vi "Store Executed Command.vi"(8 "error in (no error)":errorcluster, 10 "Completed Command":refnum<class "Command.lvclass">, 11 "Command Handler in":refnum<class "Command Handler.lvclass">) -> (0 "error out":errorcluster, 3 "Command Handler out":refnum<class "Command Handler.lvclass">)   [LabVIEW 2015, in "Command Handler.lvlib" / "Command Handler.lvclass"]
uses:
  Command Handler.lvclass
  Command Parent/Command.lvclass
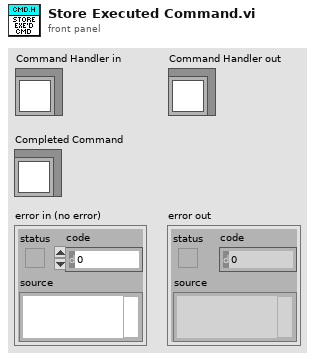
[diagram p1: front panel]
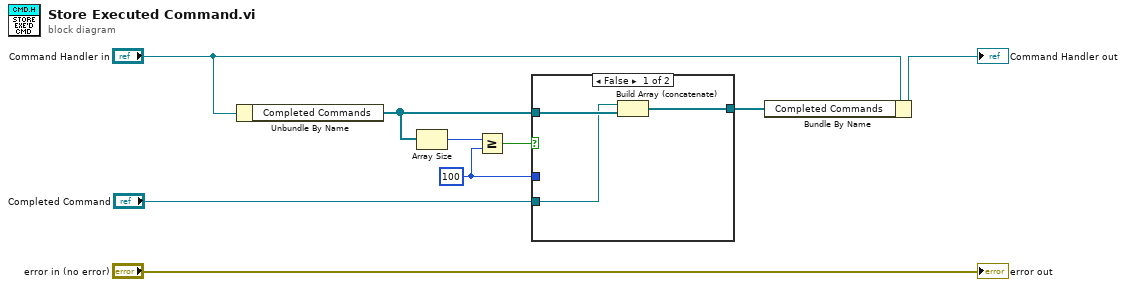
[diagram p0: block diagram]
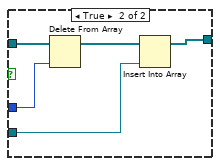
[diagram p2: hidden frame]
diagram:
  w2 = 100 ("y")
  n1 = Unbundle By Name("Command Handler in") -> ("Completed Commands"=w3:refnum<class "Command.lvclass">[])
  n2 = Array Size(array=w3) -> (size(s)=w5:i32)
  n3 = Greater Or Equal?(x=w5, y=w2) -> (x >= y?=w4:bool)
  n4 = case shown="False" w4 {
    tunnel: w3 -> [w12 w17]
    tunnel: "Completed Command" -> [w10 w14]
    tunnel: w2 -> [_ w16]
    tunnel: [w11 w13] -> w1
    frame False {
      n5 = Build Array (concatenate)(w10, w12) -> (w11:refnum<class "Command.lvclass">[])
    }
    frame True {
      n6 = Delete From Array(array=w17, index=w16) -> (array with subset deleted=w15:refnum<class "Command.lvclass">[])  [unwired: 1 in, 1 out]
      n7 = Insert Into Array(array=w15, new element=w14) -> (w13:refnum<class "Command.lvclass">[])  [unwired: 1 in]
    }
  }
  n8 = Bundle By Name(cluster="Command Handler in", "Completed Commands"=w1) -> (→"Command Handler out":refnum<class "Command Handler.lvclass">)
  "error out" <- "error in (no error)"
